vi "Start Arduino Comms.vi"(1 "Arduino comm. params.":T1={"VISA resource name"="COM9", "byte count"=64, "flow control (0:none)"=0, "stop bits (10: 1 bit)"=10, "parity (0:none)"=enum."None", "data bits (8)"=8, "termination char "=10, "Enable Termination\nChar"=TRUE, "baud rate (bps)"=115200, "timeout (ms)"=1000, "Locked"=FALSE} {"termination char" format="%02x"; "data bits (8)" min=5 max=8 step=1; "stop bits (10: 1 bit)" items=["1.0"=10, "1.5"=15, "2.0"=20]; "flow control (0:none)" items=["None", "XON/XOFF", "RTS/CTS", "XON/XOFF & RTS/CTS", "DTR/DSR", "XON/XOFF & DTR/DSR"]}) -> (0 "Error":errorcluster)   [LabVIEW 2013]
uses:
  Arduino_comm_params.ctl
  <vilib>/Instr/_visa.llb/VISA Open Access Mode.ctl
  Arduino_comms_Global.vi
  <vilib>/Instr/_visa.llb/VISA Configure Serial Port (Instr).vi
panel:
  # "(0xA = '\\n' = newline)"
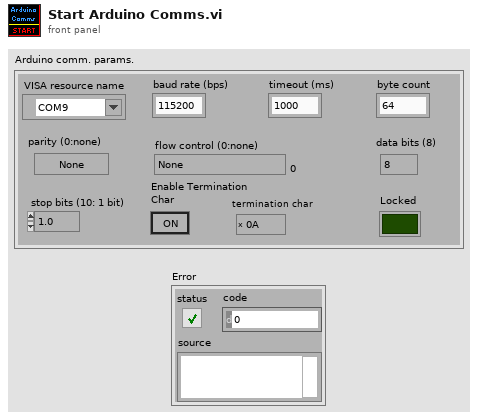
[diagram p1: front panel]
types:
  T1 = typedef "Arduino_comm_params.ctl" = cluster{"VISA resource name":refnum<visa-resource-name>, "byte count":u32, "flow control (0:none)":u16, "stop bits (10: 1 bit)":u16, "parity (0:none)":enum16{"None", "Odd", "Even", "Mark", "Space"}, "data bits (8)":u16, "termination char ":u8, "Enable Termination\nChar":bool, "baud rate (bps)":u32, "timeout (ms)":u32, "Locked":bool}
  T2 = typedef "VISA Open Access Mode.ctl" = u32
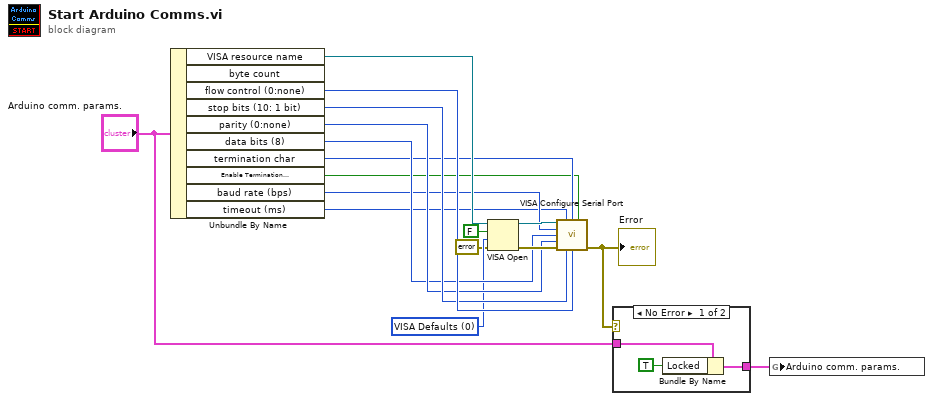
[diagram p0: block diagram]
diagram:
  w4 = T2 0 items=["VISA Defaults"=0, "Exclusive Lock"=1, "Load Configured Settings"=4] ("Access Mode")
  n1 = Unbundle By Name("Arduino comm. params.") -> ("VISA resource name"=w15:refnum<visa-resource-name>, "flow control (0:none)"=w14:u16, "stop bits (10: 1 bit)"=w13:u16, "parity (0:none)"=w12:enum16{"None", "Odd", "Even", "Mark", "Space"}, "data bits (8)"=w11:u16, "termination char"=w8:u8, "Enable Termination\nChar"=w7:bool, "baud rate (bps)"=w10:u32, "timeout (ms)"=w9:u32)  [unwired: 1 out]
  n2 = VISA Open(duplicate session (F)=FALSE, access mode=w4, error in (no error)=errorcluster {"status"=FALSE, "code"=0, "source"=""}, VISA resource name=w15) -> (VISA resource name=w17:refnum<visa-resource-name>, error out=w16:errorcluster)  [unwired: 1 in]
  n3 = call-poly "VISA Configure Serial Port"("VISA resource name"=w17, "timeout (10sec)"=w9, "termination char\n(0xA = '\\n' = LF)"=w8, "Enable Termination\nChar (T)"=w7, "baud rate (9600)"=w10, "data bits (8)"=w11, "parity (0:none)"=w12, "error in (no error)"=w16, "stop bits (10: 1 bit)"=w13, "flow control (0:none)"=w14) -> ("error out"=w1:errorcluster)  [unwired: 4 in, 1 out]
  "Error" <- w1
  n4 = case shown="No Error" w1 {
    tunnel: [w18 w21] -> w6
    tunnel: "Arduino comm. params." -> [w19 w21]
    frame No Error {
      n5 = Bundle By Name(cluster=w19, "Locked"=TRUE) -> (w18:T1)
    }
    frame Error {
    }
  }
  n6 = global write "Arduino_comms_Global.vi" "Arduino comm. params."(w6) -> ()
